vi "Pointer 2 Reference.vi"(0 "Pointer":u64 format="%.0x") -> (1 "Not A Refnum?":bool, 2 "Generic Reference":refnum<data-value>)   [LabVIEW 2013, in "Hierarchy Framework.lvlib" / "Generic.lvclass"]
uses:
  Generic.lvclass
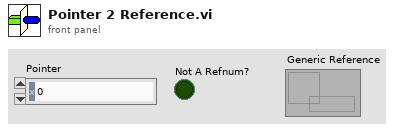
[diagram p1: front panel]
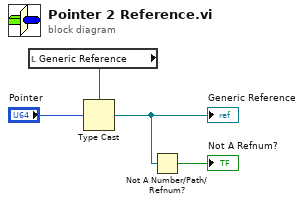
[diagram p0: block diagram]
diagram:
  n1 = local read "Generic Reference"() -> (w4:refnum<data-value>)
  n2 = Type Cast(type=w4, x="Pointer") -> (*(type *) &x=w2:refnum<data-value>)
  "Generic Reference" <- w2
  n3 = Not A Number/Path/Refnum?(number/path/refnum=w2) -> (NaN/Path/Refnum?=→"Not A Refnum?":bool)
